vi "set_pointsnumber.vi"(8 "error in (no error)":errorcluster, 11 "TrajectoryMH100122AODRAPS in":refnum<class "TrajectoryMH100122AODRAPS.lvclass">) -> (0 "error out":errorcluster, 3 "TrajectoryMH100122AODRAPS out":refnum<class "TrajectoryMH100122AODRAPS.lvclass">)   [LabVIEW 2010, in "TrajectoryMH100122AODRAPS.lvclass"]
uses:
  TrajectoryMH100122AODRAPS.lvclass
  TrajectoryMH100122AODRAPS.lvclass/TrajectoryMH100122AODRAPS.ctl
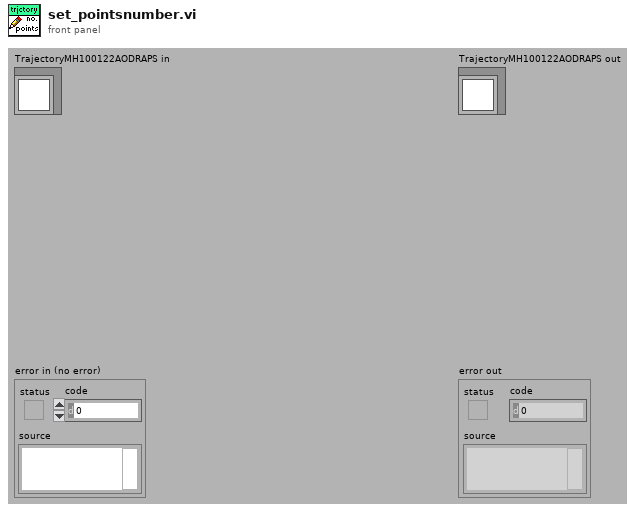
[diagram p1: front panel]
types:
  T1 = typedef "TrajectoryMH100122AODRAPS.lvclass/raps_points_cluster.ctl" = cluster{"x array":u16[], "y array":u16[], "z array":u16[], "amp array":u16[], "activation array":bool[]}
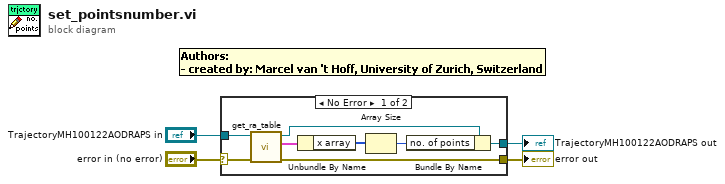
[diagram p0: block diagram]
diagram:
  n1 = case shown="No Error" "error in (no error)" {
    selector: "error in (no error)" -> [w12 w14]
    tunnel: [w11 w14] -> w3
    tunnel: [w6 w13] -> w1
    tunnel: "TrajectoryMH100122AODRAPS in" -> [w10 w13]
    frame No Error {
      n2 = call-dynamic "get_ra_table.vi"("error in (no error)"=w12, "TrajectoryMH100122AODRAPS in"=w10) -> ("error out"=w11:errorcluster, "RAPS points cluster"=w9:T1, "TrajectoryMH100122AODRAPS out"=w7:refnum<class "TrajectoryMH100122AODRAPS.lvclass">)  [unwired: 7 in]
      n3 = Unbundle By Name(w9) -> ("x array"=w8:u16[])
      n4 = Array Size(array=w8) -> (size(s)=w5:i32)
      n5 = Bundle By Name(cluster=w7, "no. of points"=w5) -> (w6:refnum<class "TrajectoryMH100122AODRAPS.lvclass">)
    }
    frame Error {
    }
  }
  "error out" <- w3
  "TrajectoryMH100122AODRAPS out" <- w1
